vi "PCO_RecorderCopyImage.vi"(0 "phRec":u64, 1 "phCam":u64, 2 "dwImgIdx":u32, 3 "wRoiX0":u16, 4 "wRoiY0":u16, 5 "wRoiX1":u16, 6 "wRoiY1":u16, 7 "error in (no error)":errorcluster {"code" format="%x"}) -> (16 "strTimestamp":T2 {"lvTimestamp" format="%<%.6X\n%x>T"}, 17 "strMetadata":T1, 20 "phRec out":u64, 21 "ErrorMessage":i32 format="%x", 22 "wImgBuf":u16[][](array[numeric]), 23 "dwImgNumber":u32, 27 "error out":errorcluster {"code" format="%x"})   [LabVIEW 2019, in "Recorder.lvlib"]
doc: "<b>Description:</b>\nThis function copies a defined ROI of the specified image from the specified camera into a preallocated buffer. If the specified image index exceeds the number of required or recorded images (depending on which value is smaller), the function will return with an error. If PCO_RECORDER_LATEST_IMAGE (see 2.10.1) is set as image index, the latest image will be copied.\n\n<b>Make sure that the transferred buffer has always at least the size of the transferred roi. Since the buffer size will not be checked internally, a buffer which is too small might crash your application.</b>\n\nIf the recorder mode is record-to-memory in conjunction with ring buffer mode and acquisition is running, it is possible that the required image will be overwritten during copy. In this case the resulting data will be unpredictable. So be careful using the function during this state.\n\nIf the mode is record-to-file and acquisition is running, the function will fail for all indices except PCO_RECORDER_LATEST_IMAGE.\n\n<b>Supported camera type:</b>\nAll cameras"
uses:
  Recorder.lvlib
  pco.sdk/Structures/Structures.lvlib
  <vilib>/Utility/miscctls.llb/LVDateTimeRec.ctl
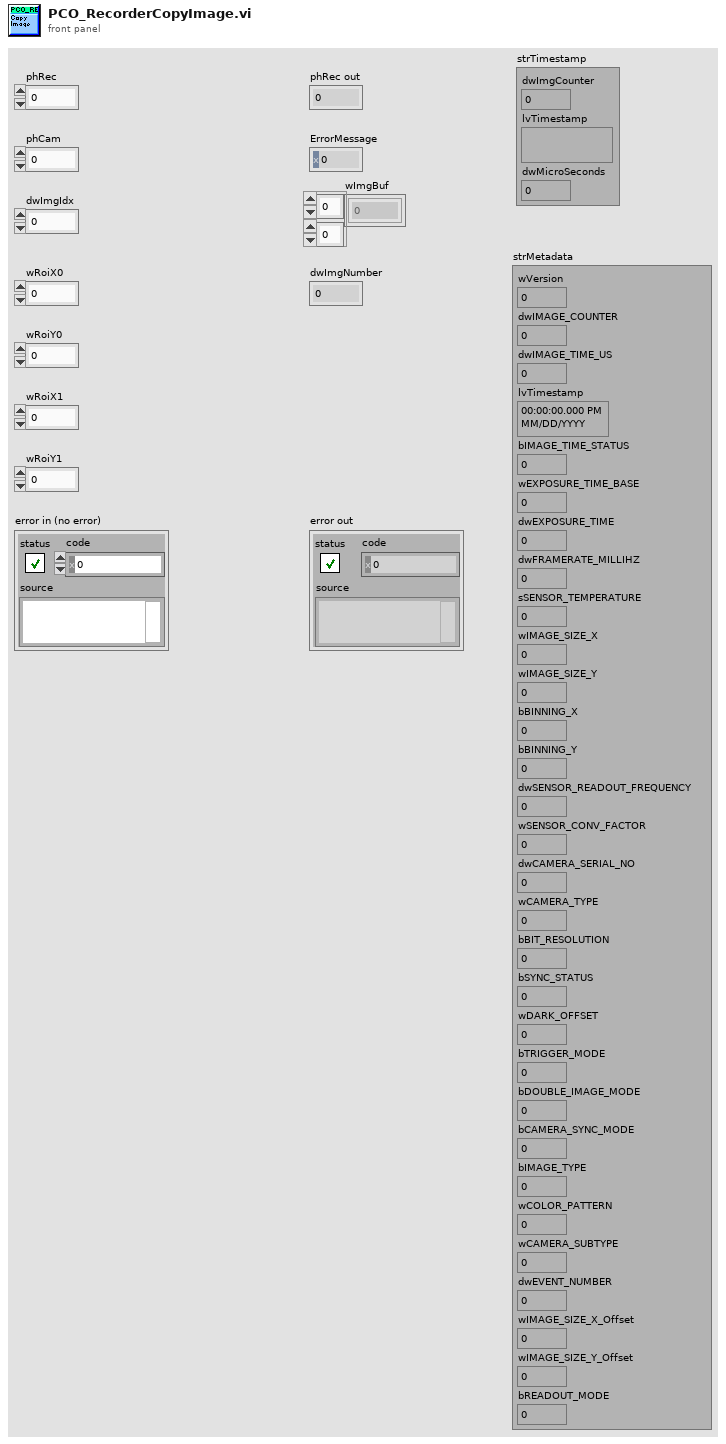
[diagram p1: front panel]
types:
  T1 = cluster{"wVersion":u16, "dwIMAGE_COUNTER":u32, "dwIMAGE_TIME_US":u32, "lvTimestamp":timestamp, "bIMAGE_TIME_STATUS":u8, "wEXPOSURE_TIME_BASE":u16, "dwEXPOSURE_TIME":u32, "dwFRAMERATE_MILLIHZ":u32, "sSENSOR_TEMPERATURE":i16, "wIMAGE_SIZE_X":u16, "wIMAGE_SIZE_Y":u16, "bBINNING_X":u8, "bBINNING_Y":u8, "dwSENSOR_READOUT_FREQUENCY":u32, "wSENSOR_CONV_FACTOR":u16, "dwCAMERA_SERIAL_NO":u32, "wCAMERA_TYPE":u16, "bBIT_RESOLUTION":u8, "bSYNC_STATUS":u8, "wDARK_OFFSET":u16, "bTRIGGER_MODE":u8, "bDOUBLE_IMAGE_MODE":u8, "bCAMERA_SYNC_MODE":u8, "bIMAGE_TYPE":u8, "wCOLOR_PATTERN":u16, "wCAMERA_SUBTYPE":u16, "dwEVENT_NUMBER":u32, "wIMAGE_SIZE_X_Offset":u16, "wIMAGE_SIZE_Y_Offset":u16, "bREADOUT_MODE":u8}
  T2 = cluster{"dwImgCounter":u32, "lvTimestamp":timestamp, "dwMicroSeconds":u32}
  T3 = enum16{"big-endian, network order", "native, host order", "little-endian"}
  T4 = typedef "LVDateTimeRec.ctl" = cluster{"fractional second":dbl, "second":i32, "minute":i32, "hour":i32, "day of month":i32, "month":i32, "year":i32, "day of week":i32, "day of year":i32, "DST":i32}
  T5 = cluster{"wSize":u16, "dwImgCounter":u32, "wYear":u16, "wMonth":u16, "wDay":u16, "wHour":u16, "wMinute":u16, "wSecond":u16, "dwMicroSeconds":u32}
  T6 = cluster{"wSize":u16, "wVersion":u16, "bIMAGE_COUNTER_BCD":cluster{u8, u8, u8, u8}, "bIMAGE_TIME_US_BCD":cluster{u8, u8, u8}, "bIMAGE_TIME_SEC_BCD":u8, "bIMAGE_TIME_MIN_BCD":u8, "bIMAGE_TIME_HOUR_BCD":u8, "bIMAGE_TIME_DAY_BCD":u8, "bIMAGE_TIME_MON_BCD":u8, "bIMAGE_TIME_YEAR_BCD":u8, "bIMAGE_TIME_STATUS":u8, "wEXPOSURE_TIME_BASE":u16, "dwEXPOSURE_TIME":u32, "dwFRAMERATE_MILLIHZ":u32, "sSENSOR_TEMPERATURE":i16, "wIMAGE_SIZE_X":u16, "wIMAGE_SIZE_Y":u16, "bBINNING_X":u8, "bBINNING_Y":u8, "dwSENSOR_READOUT_FREQUENCY":u32, "wSENSOR_CONV_FACTOR":u16, "dwCAMERA_SERIAL_NO":u32, "wCAMERA_TYPE":u16, "bBIT_RESOLUTION":u8, "bSYNC_STATUS":u8, "wDARK_OFFSET":u16, "bTRIGGER_MODE":u8, "bDOUBLE_IMAGE_MODE":u8, "bCAMERA_SYNC_MODE":u8, "bIMAGE_TYPE":u8, "wCOLOR_PATTERN":u16, "wCAMERA_SUBTYPE":u16, "dwEVENT_NUMBER":u32, "wIMAGE_SIZE_X_Offset":u16, "wIMAGE_SIZE_Y_Offset":u16, "bREADOUT_MODE":u8}
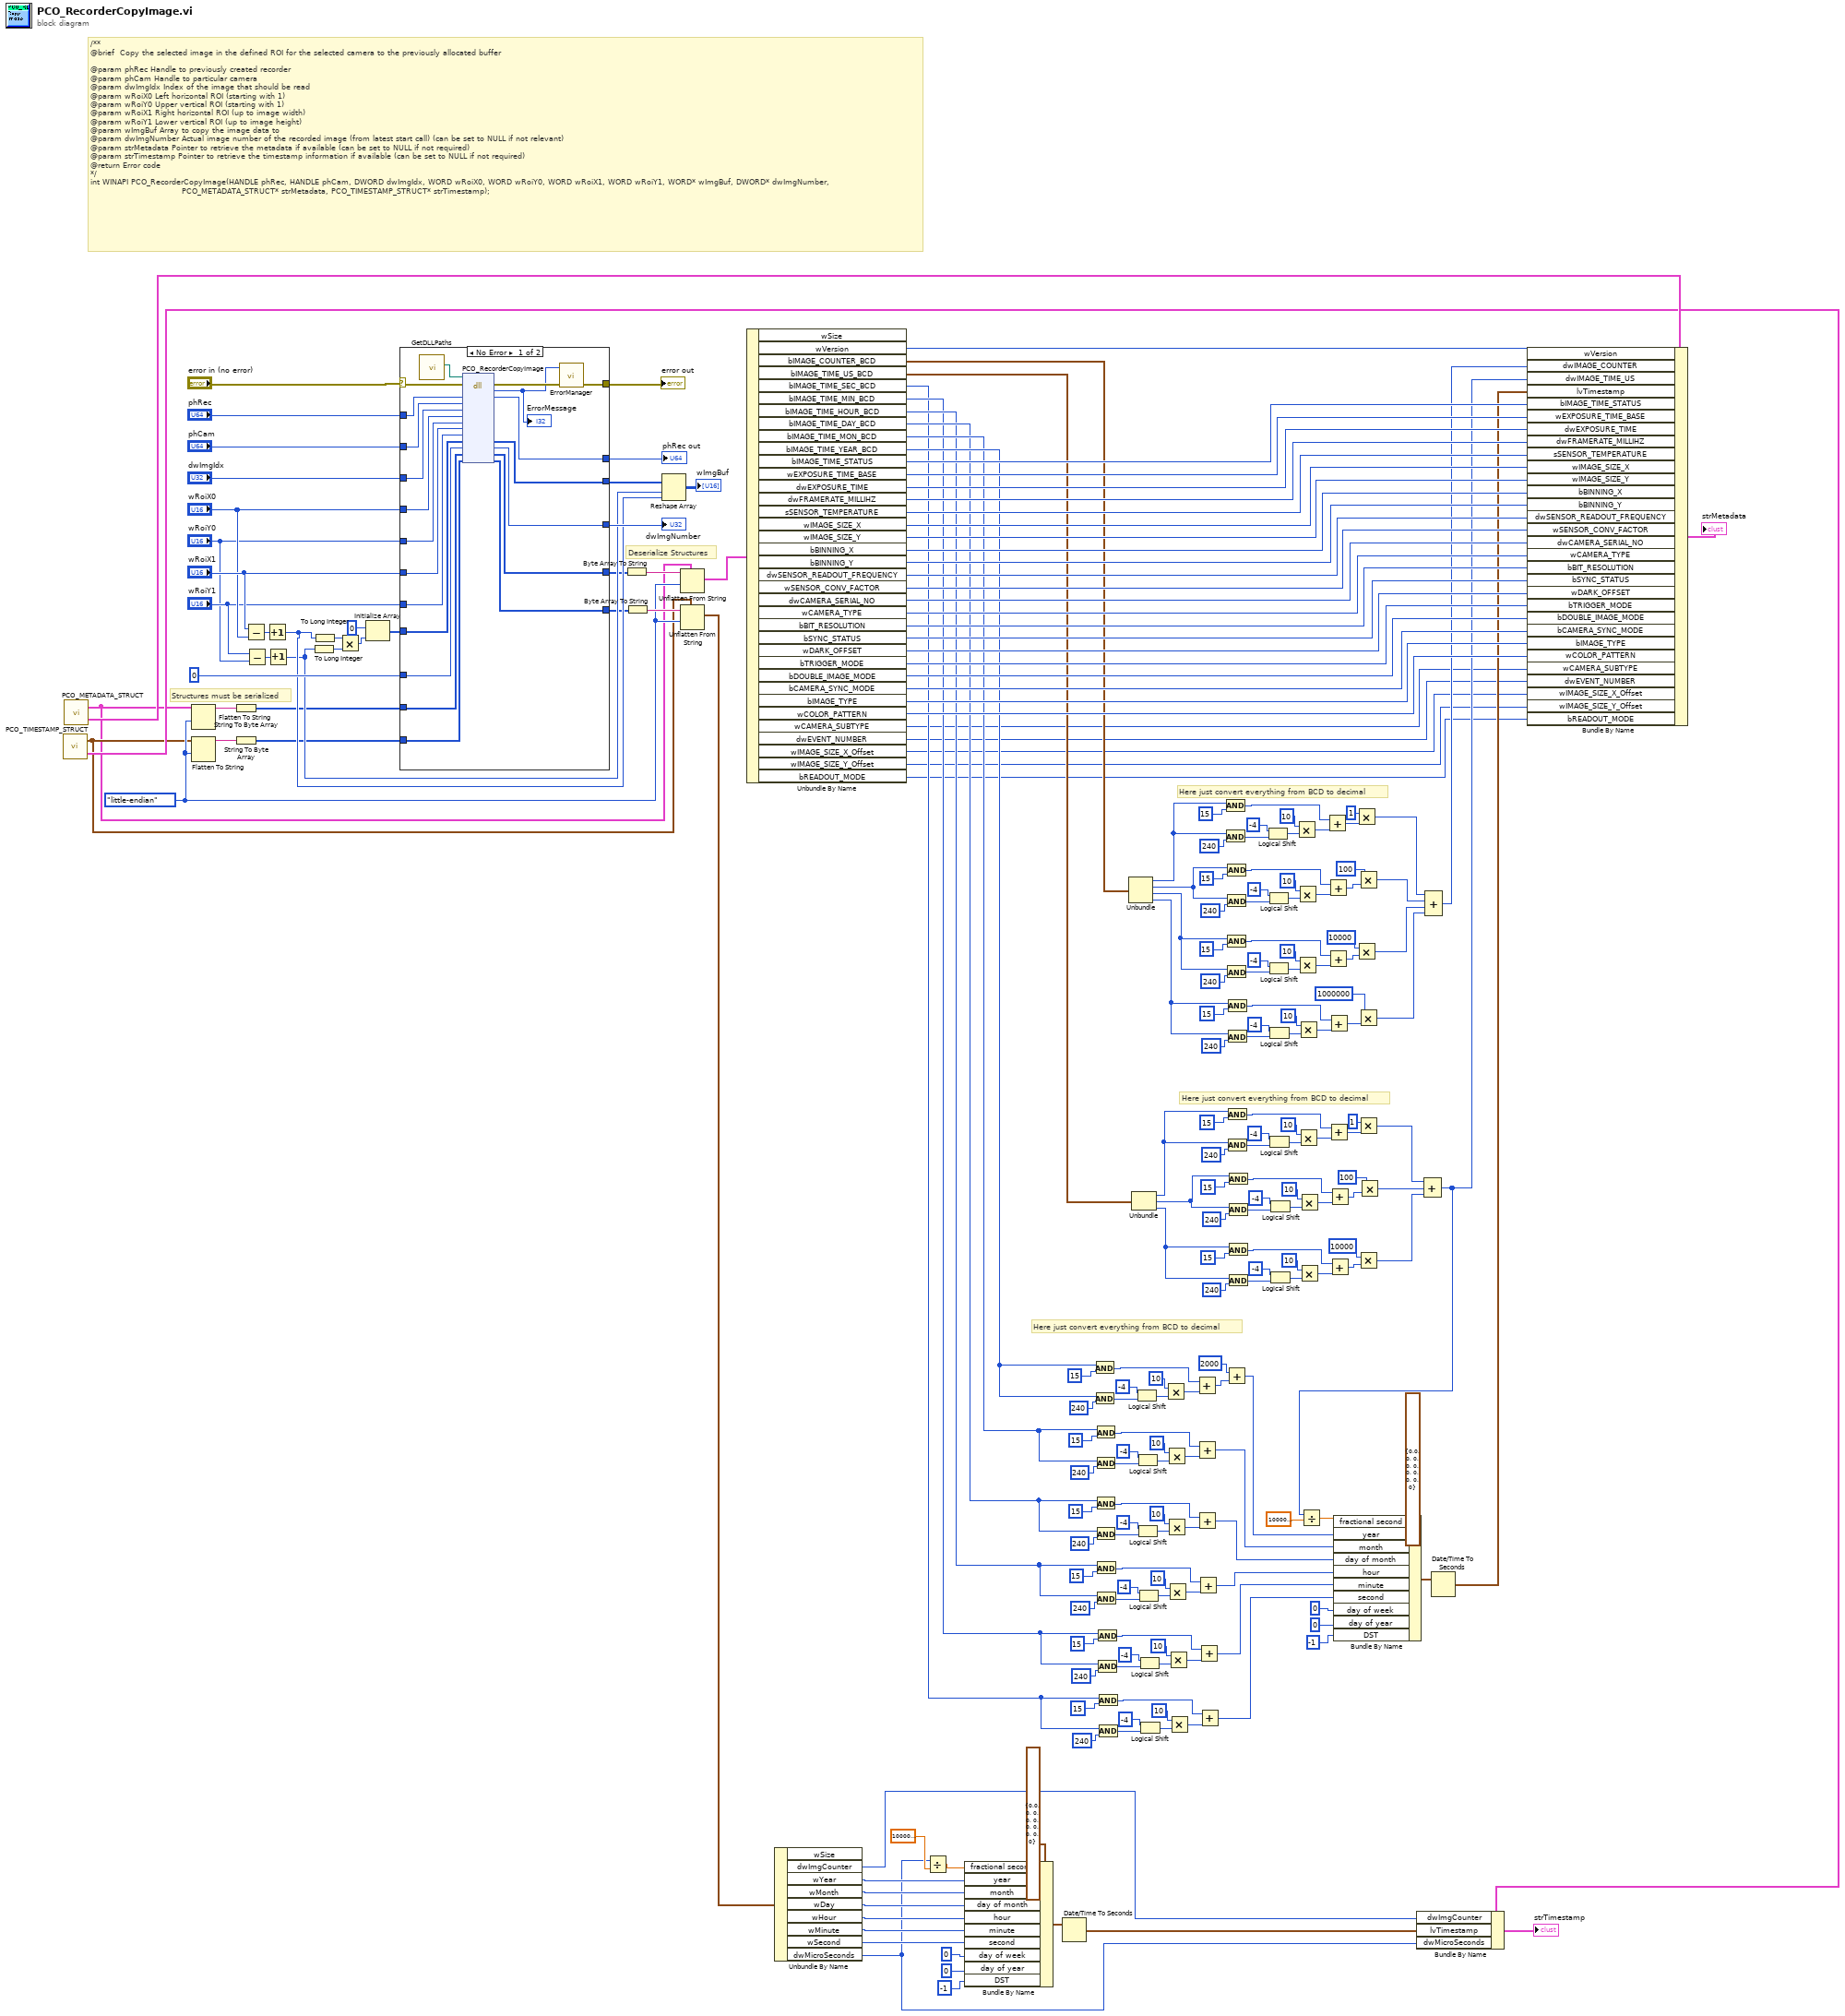
[diagram p0: block diagram]
diagram:
  w18 = T3."little-endian" ("Byte-Reihenfolge (0:Big-Endian, Netzwerkreihenfolge)")
  # "Deserialize Structures"
  # "Structures must be serialized"
  # "Here just convert everything from BCD to decimal"
  # "Here just convert everything from BCD to decimal"
  # "Here just convert everything from BCD to decimal"
  # "/**\n@brief \tCopy the selected image in the defined ROI for the selected camera to the previously allocated buffer\n\n@param phRec Handle to previously created recorder\n@param phCam Handle to particular camera\n@param dwImgIdx Index of the image that should be read\n@param wRoiX0 Left horizontal ROI (starting with 1)\n@param wRoiY0 Upper vertical ROI (starting with 1)\n@param wRoiX1 Right horizontal ROI (up to image width)\n@param wRoiY1 Lower vertical ROI (up to image height)\n@param wImgBuf Array to copy the image data to\n@param dwImgNumber Actual image number of the recorded image (from latest start call) (can be set to NULL if not relevant)\n@param strMetadata Pointer to retrieve the metadata if available (can be set to NULL if not required)\n@param strTimestamp Pointer to retrieve the timestamp information if available (can be set to NULL if not required)\n@return Error code\n*/\nint WINAPI PCO_RecorderCopyImage(HANDLE phRec, HANDLE phCam, DWORD dwImgIdx, WORD wRoiX0, WORD wRoiY0, WORD wRoiX1, WORD wRoiY1, WORD* wImgBuf, DWORD* dwImgNumber, \n                                 PCO_METADATA_STRUCT* strMetadata, PCO_TIMESTAMP_STRUCT* strTimestamp);"
  n1 = call "PCO_TIMESTAMP_STRUCT.vi"() -> ("PCO_TIMESTAMP_STRUCT"=w219:T2, "PCO_TIMESTAMP_STRUCT_Raw"=w17:T5)  [unwired: 4 in, 2 out]
  n2 = call "PCO_METADATA_STRUCT.vi"() -> ("PCO_METADATA_STRUCT"=w224:T1, "PCO_METADATA_STRUCT_Raw"=w16:T6)  [unwired: 4 in, 2 out]
  n3 = Flatten To String(anything=w16, byte order (0:big-endian, network order)=w18) -> (data string=w26:string)  [unwired: 2 in, 2 out]
  n4 = Flatten To String(anything=w17, byte order (0:big-endian, network order)=w18) -> (data string=w28:string)  [unwired: 2 in, 2 out]
  n5 = String To Byte Array(string=w26) -> (unsigned byte array=w25:u8[])
  n6 = String To Byte Array(string=w28) -> (unsigned byte array=w27:u8[])
  n7 = Subtract(x="wRoiX1", y="wRoiX0") -> (x-y=w229:u16)
  n8 = Subtract(x="wRoiY1", y="wRoiY0") -> (x-y=w226:u16)
  n9 = Increment(x=w229) -> (x+1=w30:u16)
  n10 = Increment(x=w226) -> (x+1=w29:u16)
  n11 = To Long Integer(number=w29) -> (32bit integer=w32:i32)
  n12 = To Long Integer(number=w30) -> (32bit integer=w31:i32)
  n13 = Multiply(x=w31, y=w32) -> (x*y=w225:i32)
  n14 = Initialize Array(u16 0 ("element"), w225) -> (w237:u16[])
  n15 = case shown="No Error" "error in (no error)" {
    selector: "error in (no error)" -> [w249 w268]
    tunnel: "phRec" -> [w262 w267]
    tunnel: [w261 w267] -> w240
    tunnel: "phCam" -> [w260 _]
    tunnel: "dwImgIdx" -> [w259 _]
    tunnel: "wRoiX0" -> [w258 _]
    tunnel: "wRoiY0" -> [w257 _]
    tunnel: "wRoiX1" -> [w256 _]
    tunnel: "wRoiY1" -> [w255 _]
    tunnel: w237 -> [w254 w266]
    tunnel: [w253 w266] -> w34
    tunnel: [w252 w265] -> w235
    tunnel: [w251 w264] -> w24
    tunnel: [w250 w263] -> w23
    tunnel: [w248 w268] -> w234
    tunnel: w27 -> [w245 w263]
    tunnel: w25 -> [w244 w264]
    tunnel: u32 0 ("dwImgNumber") -> [w243 w265]
    frame No Error {
      n16 = call "GetDLLPaths.vi"() -> ("PCO_Recorder_Path"=w242:path)  [unwired: 8 in, 3 out]
      n17 = dll-call lib="?" fn="PCO_RecorderCopyImage"(path in=w242, error in=w249, "phRec"=w262, "phCam"=w260, "dwImgIdx"=w259, "wRoiX0"=w258, "wRoiY0"=w257, "wRoiX1"=w256, "wRoiY1"=w255, "wImgBuf"=w254, "dwImgNumber"=w243, "strMetadata"=w244, "strTimestamp"=w245) -> (error out=w247:errorcluster, "return type"=w246:i32, "phRec"=w261:u64, "wImgBuf"=w253:u16[], "dwImgNumber"=w252:u32, "strMetadata"=w251:u8[], "strTimestamp"=w250:u8[])  [unwired: 7 in, 1 out]
      "ErrorMessage" <- w246
      n18 = call "ErrorManager.vi"("error in (no error)"=w247, "error code"=w246) -> ("error out"=w248:errorcluster)  [unwired: 2 in, 1 out]
    }
    frame Error {
    }
  }
  "phRec out" <- w240
  "dwImgNumber" <- w235
  "error out" <- w234
  n19 = Byte Array To String(unsigned byte array=w24) -> (string=w22:string)
  n20 = Byte Array To String(unsigned byte array=w23) -> (string=w21:string)
  n21 = Reshape Array(w34, w29, w30) -> (→"wImgBuf":u16[][])
  n22 = Unflatten From String(type=w16, binary string=w22, byte order (0:big-endian, network order)=w18) -> (value=w20:T6)  [unwired: 2 in, 2 out]
  n23 = Unflatten From String(type=w17, binary string=w21, byte order (0:big-endian, network order)=w18) -> (value=w19:T5)  [unwired: 2 in, 2 out]
  n24 = Unbundle By Name(w20) -> ("wVersion"=w223:u16, "bIMAGE_COUNTER_BCD"=w121:cluster{u8, u8, u8, u8}, "bIMAGE_TIME_US_BCD"=w43:cluster{u8, u8, u8}, "bIMAGE_TIME_SEC_BCD"=w133:u8, "bIMAGE_TIME_MIN_BCD"=w134:u8, "bIMAGE_TIME_HOUR_BCD"=w135:u8, "bIMAGE_TIME_DAY_BCD"=w136:u8, "bIMAGE_TIME_MON_BCD"=w137:u8, "bIMAGE_TIME_YEAR_BCD"=w182:u8, "bIMAGE_TIME_STATUS"=w204:u8, "wEXPOSURE_TIME_BASE"=w203:u16, "dwEXPOSURE_TIME"=w202:u32, "dwFRAMERATE_MILLIHZ"=w201:u32, "sSENSOR_TEMPERATURE"=w200:i16, "wIMAGE_SIZE_X"=w199:u16, "wIMAGE_SIZE_Y"=w198:u16, "bBINNING_X"=w197:u8, "bBINNING_Y"=w196:u8, "dwSENSOR_READOUT_FREQUENCY"=w195:u32, "wSENSOR_CONV_FACTOR"=w194:u16, "dwCAMERA_SERIAL_NO"=w193:u32, "wCAMERA_TYPE"=w192:u16, "bBIT_RESOLUTION"=w191:u8, "bSYNC_STATUS"=w190:u8, "wDARK_OFFSET"=w189:u16, "bTRIGGER_MODE"=w188:u8, "bDOUBLE_IMAGE_MODE"=w187:u8, "bCAMERA_SYNC_MODE"=w186:u8, "bIMAGE_TYPE"=w185:u8, "wCOLOR_PATTERN"=w184:u16, "wCAMERA_SUBTYPE"=w6:u16, "dwEVENT_NUMBER"=w5:u32, "wIMAGE_SIZE_X_Offset"=w4:u16, "wIMAGE_SIZE_Y_Offset"=w3:u16, "bREADOUT_MODE"=w1:u8)  [unwired: 1 out]
  n25 = Unbundle By Name(w19) -> ("dwImgCounter"=w206:u32, "wYear"=w208:u16, "wMonth"=w209:u16, "wDay"=w210:u16, "wHour"=w211:u16, "wMinute"=w212:u16, "wSecond"=w213:u16, "dwMicroSeconds"=w14:u32)  [unwired: 1 out]
  n26 = Divide(x=w14, y=1000000.0 ("fractional second")) -> (x/y=w13:dbl)
  n27 = Bundle By Name(cluster=T4 {"fractional second"=0.0, "second"=0, "minute"=0, "hour"=0, "day of month"=0, "month"=0, "year"=0, "day of week"=0, "day of year"=0, "DST"=0} ("date time rec"), "fractional second"=w13, "year"=w208, "month"=w209, "day of month"=w210, "hour"=w211, "minute"=w212, "second"=w213, "day of week"=0, "day of year"=0, "DST"=-1) -> (w218:T4)
  n28 = Date/Time To Seconds(2:w218) -> (0:w207:timestamp)  [unwired: 1 in]
  n29 = And(x=w182, y=u8 15) -> (x .and. y?=w178:u8)
  n30 = And(x=w182, y=u8 240) -> (x .and. y?=w220:u8)
  n31 = And(x=w137, y=u8 15) -> (x .and. y?=w177:u8)
  n32 = And(x=w137, y=u8 240) -> (x .and. y?=w172:u8)
  n33 = And(x=w136, y=u8 15) -> (x .and. y?=w161:u8)
  n34 = And(x=w136, y=u8 240) -> (x .and. y?=w156:u8)
  n35 = And(x=w135, y=u8 15) -> (x .and. y?=w162:u8)
  n36 = And(x=w135, y=u8 240) -> (x .and. y?=w167:u8)
  n37 = And(x=w134, y=u8 15) -> (x .and. y?=w146:u8)
  n38 = And(x=w134, y=u8 240) -> (x .and. y?=w151:u8)
  n39 = And(x=w133, y=u8 15) -> (x .and. y?=w145:u8)
  n40 = And(x=w133, y=u8 240) -> (x .and. y?=w140:u8)
  n41 = Unbundle(w121) -> (w51:u8, w50:u8, w49:u8, w48:u8)
  n42 = Unbundle(w43) -> (w42:u8, w41:u8, w40:u8)
  n43 = Logical Shift(y=i16 -4, x=w220) -> (x << y=w181:u8)
  n44 = Logical Shift(y=i16 -4, x=w172) -> (x << y=w174:u8)
  n45 = Logical Shift(y=i16 -4, x=w156) -> (x << y=w158:u8)
  n46 = Logical Shift(y=i16 -4, x=w167) -> (x << y=w165:u8)
  n47 = Logical Shift(y=i16 -4, x=w151) -> (x << y=w149:u8)
  n48 = Logical Shift(y=i16 -4, x=w140) -> (x << y=w142:u8)
  n49 = Multiply(x=u8 10, y=w181) -> (x*y=w179:u8)
  n50 = Multiply(x=u8 10, y=w174) -> (x*y=w176:u8)
  n51 = Multiply(x=u8 10, y=w158) -> (x*y=w160:u8)
  n52 = Multiply(x=u8 10, y=w165) -> (x*y=w163:u8)
  n53 = Multiply(x=u8 10, y=w149) -> (x*y=w147:u8)
  n54 = Multiply(x=u8 10, y=w142) -> (x*y=w144:u8)
  n55 = Add(x=w178, y=w179) -> (x+y=w12:u8)
  n56 = Add(x=w177, y=w176) -> (x+y=w127:u8)
  n57 = Add(x=w161, y=w160) -> (x+y=w126:u8)
  n58 = Add(x=w162, y=w163) -> (x+y=w125:u8)
  n59 = Add(x=w146, y=w147) -> (x+y=w124:u8)
  n60 = Add(x=w145, y=w144) -> (x+y=w123:u8)
  n61 = And(x=w51, y=u8 15) -> (x .and. y?=w96:u8)
  n62 = And(x=w51, y=u8 240) -> (x .and. y?=w91:u8)
  n63 = And(x=w50, y=u8 15) -> (x .and. y?=w97:u8)
  n64 = And(x=w50, y=u8 240) -> (x .and. y?=w102:u8)
  n65 = And(x=w49, y=u8 15) -> (x .and. y?=w113:u8)
  n66 = And(x=w49, y=u8 240) -> (x .and. y?=w118:u8)
  n67 = Add(x=2000, y=w12) -> (x+y=w10:i32)
  n68 = And(x=w48, y=u8 15) -> (x .and. y?=w112:u8)
  n69 = And(x=w48, y=u8 240) -> (x .and. y?=w107:u8)
  n70 = And(x=w42, y=u8 15) -> (x .and. y?=w67:u8)
  n71 = And(x=w42, y=u8 240) -> (x .and. y?=w72:u8)
  n72 = And(x=w41, y=u8 15) -> (x .and. y?=w66:u8)
  n73 = And(x=w41, y=u8 240) -> (x .and. y?=w61:u8)
  n74 = And(x=w40, y=u8 15) -> (x .and. y?=w58:u8)
  n75 = And(x=w40, y=u8 240) -> (x .and. y?=w53:u8)
  n76 = Logical Shift(y=i16 -4, x=w91) -> (x << y=w93:u8)
  n77 = Logical Shift(y=i16 -4, x=w102) -> (x << y=w100:u8)
  n78 = Logical Shift(y=i16 -4, x=w118) -> (x << y=w116:u8)
  n79 = Logical Shift(y=i16 -4, x=w107) -> (x << y=w109:u8)
  n80 = Logical Shift(y=i16 -4, x=w72) -> (x << y=w70:u8)
  n81 = Logical Shift(y=i16 -4, x=w61) -> (x << y=w63:u8)
  n82 = Logical Shift(y=i16 -4, x=w53) -> (x << y=w55:u8)
  n83 = Multiply(x=u8 10, y=w93) -> (x*y=w95:u8)
  n84 = Multiply(x=u8 10, y=w100) -> (x*y=w98:u8)
  n85 = Multiply(x=u8 10, y=w116) -> (x*y=w114:u8)
  n86 = Multiply(x=u8 10, y=w109) -> (x*y=w111:u8)
  n87 = Multiply(x=u8 10, y=w70) -> (x*y=w68:u8)
  n88 = Multiply(x=u8 10, y=w63) -> (x*y=w65:u8)
  n89 = Multiply(x=u8 10, y=w55) -> (x*y=w57:u8)
  n90 = Add(x=w96, y=w95) -> (x+y=w85:u8)
  n91 = Add(x=w97, y=w98) -> (x+y=w88:u8)
  n92 = Add(x=w113, y=w114) -> (x+y=w87:u8)
  n93 = Add(x=w112, y=w111) -> (x+y=w86:u8)
  n94 = Add(x=w67, y=w68) -> (x+y=w77:u8)
  n95 = Add(x=w66, y=w65) -> (x+y=w75:u8)
  n96 = Add(x=w58, y=w57) -> (x+y=w76:u8)
  n97 = Multiply(x=u32 1, y=w85) -> (x*y=w47:u32)
  n98 = Multiply(x=u32 10000, y=w87) -> (x*y=w45:u32)
  n99 = Multiply(x=u32 100, y=w88) -> (x*y=w46:u32)
  n100 = Multiply(x=u32 1000000, y=w86) -> (x*y=w44:u32)
  n101 = Multiply(x=u32 1, y=w77) -> (x*y=w38:u32)
  n102 = Multiply(x=u32 10000, y=w76) -> (x*y=w36:u32)
  n103 = Multiply(x=u32 100, y=w75) -> (x*y=w37:u32)
  n104 = Bundle By Name(cluster=w219, "dwImgCounter"=w206, "lvTimestamp"=w207, "dwMicroSeconds"=w14) -> (→"strTimestamp":T2)
  n105 = Compound Arithmetic op=ADD(w38, w37, w36) -> (w8:u32)
  n106 = Divide(x=w8, y=1000000.0 ("fractional second")) -> (x/y=w7:dbl)
  n107 = Bundle By Name(cluster=T4 {"fractional second"=0.0, "second"=0, "minute"=0, "hour"=0, "day of month"=0, "month"=0, "year"=0, "day of week"=0, "day of year"=0, "DST"=0} ("date time rec"), "fractional second"=w7, "year"=w10, "month"=w127, "day of month"=w126, "hour"=w125, "minute"=w124, "second"=w123, "day of week"=0, "day of year"=0, "DST"=-1) -> (w128:T4)
  n108 = Compound Arithmetic op=ADD(w47, w46, w45, w44) -> (w35:u32)
  n109 = Date/Time To Seconds(2:w128) -> (0:w122:timestamp)  [unwired: 1 in]
  n110 = Bundle By Name(cluster=w224, "wVersion"=w223, "dwIMAGE_COUNTER"=w35, "dwIMAGE_TIME_US"=w8, "lvTimestamp"=w122, "bIMAGE_TIME_STATUS"=w204, "wEXPOSURE_TIME_BASE"=w203, "dwEXPOSURE_TIME"=w202, "dwFRAMERATE_MILLIHZ"=w201, "sSENSOR_TEMPERATURE"=w200, "wIMAGE_SIZE_X"=w199, "wIMAGE_SIZE_Y"=w198, "bBINNING_X"=w197, "bBINNING_Y"=w196, "dwSENSOR_READOUT_FREQUENCY"=w195, "wSENSOR_CONV_FACTOR"=w194, "dwCAMERA_SERIAL_NO"=w193, "wCAMERA_TYPE"=w192, "bBIT_RESOLUTION"=w191, "bSYNC_STATUS"=w190, "wDARK_OFFSET"=w189, "bTRIGGER_MODE"=w188, "bDOUBLE_IMAGE_MODE"=w187, "bCAMERA_SYNC_MODE"=w186, "bIMAGE_TYPE"=w185, "wCOLOR_PATTERN"=w184, "wCAMERA_SUBTYPE"=w6, "dwEVENT_NUMBER"=w5, "wIMAGE_SIZE_X_Offset"=w4, "wIMAGE_SIZE_Y_Offset"=w3, "bREADOUT_MODE"=w1) -> (→"strMetadata":T1)
